vi "DELETE Z Position Set-point.vi"   [LabVIEW 2013]
uses:
  Action.ctl
  Set Points FGV Selector.ctl
types:
  T1 = typedef "Set Points FGV Selector.ctl" = enum16{"X Position", "Y Position", "Z Position"}
  T2 = typedef "Action.ctl" = enum16{"GET", "PUT", "DELETE"}
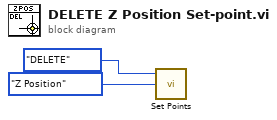
[diagram p0: block diagram]
diagram:
  n1 = call "Set Points.vi"("Set Points FGV Selector"=Set_Points_FGV_Selector."Z Position", "Action"=Action."DELETE") -> ()  [unwired: 1 in, 1 out]
